vi "5492_TalonDriveTrainPID.vi"(0 "P Left":dbl, 1 "I Left":dbl, 2 "D Left":dbl, 3 "P Right":dbl, 4 "I Right":dbl, 5 "D Right":dbl) -> (14 "RobotDriveDevRef":T1={"DevStatus"={"status"=FALSE, "code"=0, "source"=""}, "Motors[]"=[], "Square Inputs"=FALSE, "Max Output"=1.0})   [LabVIEW 2017]
uses:
  <vilib>/Rock Robotics/WPI/RobotDrive/WPI_RobotDriveDevRef.ctl
  <vilib>/Rock Robotics/WPI/MotorControl/WPI_MotorControlDeviceRef.ctl
  <vilib>/Rock Robotics/WPI/MotorControl/WPI_MotorControlType.ctl
  <vilib>/Rock Robotics/SystemInterfaces/DIO/FPGA_DIOPWMChannel.ctl
  <vilib>/Rock Robotics/WPI/PWM/WPI_PWMDeadband.ctl
  <vilib>/Rock Robotics/SystemInterfaces/DIO/FPGA_DIOChannel.ctl
  5492_WPI_RobotDriveMotorSelectorEnum.ctl
  Public/Documents/Cross The Road Electronics/Phoenix-LabVIEW/Motor Controller/Controls/CTRE_Phoenix_MotorControl_FeedbackDevice.ctl
  <vilib>/Rock Robotics/WPI/Utilities/WPI_GetSetVariantRefNum.vi
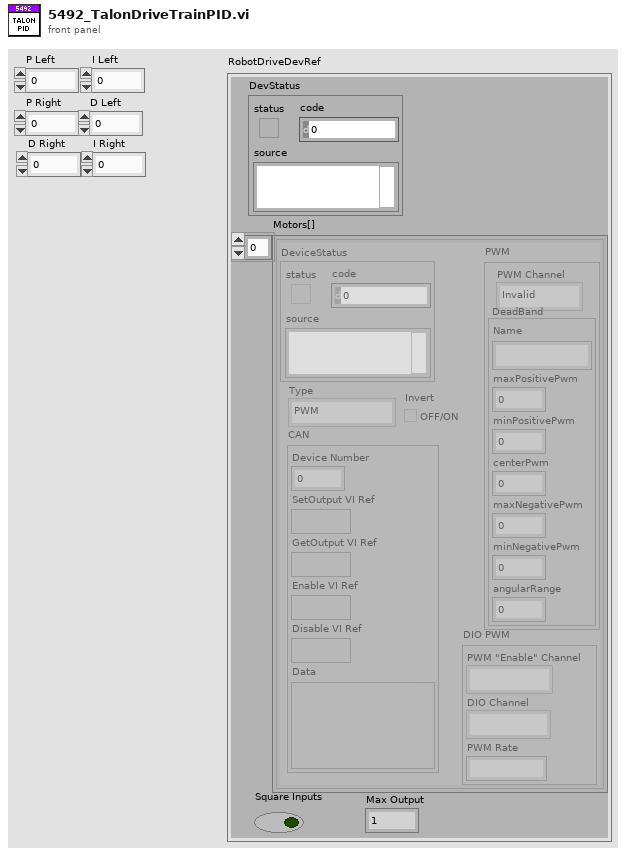
[diagram p1: front panel]
types:
  T1 = typedef "WPI_RobotDriveDevRef.ctl" = cluster{"DevStatus":errorcluster, "Motors[]":T2[], "Square Inputs":bool, "Max Output":dbl}
  T2 = typedef "WPI_MotorControlDeviceRef.ctl" = cluster{"DeviceStatus":errorcluster, "Type":T3, "PWM":cluster{"PWM Channel":T4, "DeadBand":T5}, "CAN":cluster{"Device Number":u8, "SetOutput VI Ref":variant, "GetOutput VI Ref":variant, "Enable VI Ref":variant, "Disable VI Ref":variant, "Data":variant}, "Invert":bool, "DIO PWM":cluster{"PWM \"Enable\" Channel":T4, "DIOChannel":T6, "PWM Rate":dbl}}
  T3 = typedef "WPI_MotorControlType.ctl" = enum16{"PWM", "CAN", "DIO PWM"}
  T4 = typedef "FPGA_DIOPWMChannel.ctl" = enum8{"PWM 0", "PWM 1", "PWM 2", "PWM 3", "PWM 4", "PWM 5", "PWM 6", "PWM 7", "PWM 8", "PWM 9", "PWM MXP 0", "PWM MXP 1", "PWM MXP 2", "PWM MXP 3", "PWM MXP 4", "PWM MXP 5", "PWM MXP 6", "PWM MXP 7", "PWM MXP 8", "PWM MXP 9", "Invalid"}
  T5 = typedef "WPI_PWMDeadband.ctl" = cluster{"Name":string, "maxPositivePwm":i32, "minPositivePwm":i32, "centerPwm":i32, "maxNegativePwm":i32, "minNegativePwm":i32, "angularRange":u16}
  T6 = typedef "FPGA_DIOChannel.ctl" = enum8{"DIO 0", "DIO 1", "DIO 2", "DIO 3", "DIO 4", "DIO 5", "DIO 6", "DIO 7", "DIO 8", "DIO 9", "DIO MXP 0", "DIO MXP 1", "DIO MXP 2", "DIO MXP 3", "DIO MXP 4", "DIO MXP 5", "DIO MXP 6", "DIO MXP 7", "DIO MXP 8", "DIO MXP 9", "DIO MXP 10", "DIO MXP 11", "DIO MXP 12", "DIO MXP 13", "DIO MXP 14", "DIO MXP 15", "SPI Port CS1", "SPI Port CS2", "SPI Port CS3", "SPI Port MISO", "SPI Port MOSI", "Invalid"}
  T7 = typedef "CTRE_Phoenix_MotorControl_FeedbackDevice.ctl" = i8
  T8 = typedef "5492_WPI_RobotDriveMotorSelectorEnum.ctl" = enum16{"Front left motor", "Front right motor"}
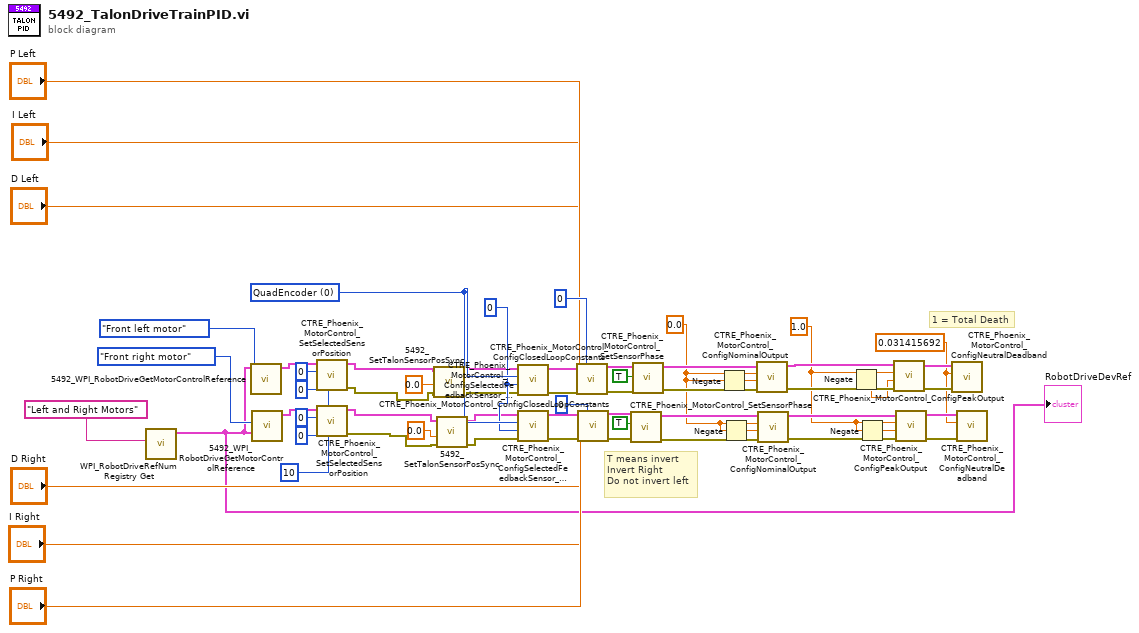
[diagram p0: block diagram]
diagram:
  w3 = 0.031415692 ("Percent Deadband")
  w11 = 0.0 ("Forward Nominal Percent Output")
  w12 = 1.0 ("Forward Peak Percent Output")
  w37 = u32 10 ("timeoutMs")
  w56 = 0 ("pidLoopIdx")
  w57 = T7 0 items=["None"=-1, "QuadEncoder"=0, "Analog"=2, "Tachometer"=4, "Pulse Width Encoded Position"=8, "Sensor Sum (S0 + S1)"=9, "Sensor Difference (D0 - D1)"=10, "Remote Source 0"=11, "Remote Source 1"=12, "Software Emulated"=15] ("Feedback Device")
  # "1 = Total Death"
  # "T means invert\nInvert Right\nDo not invert left"
  n1 = call <vilib>:"WPI_RobotDriveRefNum Registry Get.vi"("refnum name"="Left and Right Motors") -> ("RobotDriveDevRef"=w2:T1)  [unwired: 1 in, 9 out]
  "RobotDriveDevRef" <- w2
  n2 = call "5492_WPI_RobotDriveGetMotorControlReference.vi"("MotorIndex"=5492_WPI_RobotDriveMotorSelectorEnum."Front left motor", "RobotDriveDevRef"=w2) -> ("MotorControlDeviceRef"=w43:T2)  [unwired: 9 out]
  n3 = call "5492_WPI_RobotDriveGetMotorControlReference.vi"("MotorIndex"=5492_WPI_RobotDriveMotorSelectorEnum."Front right motor", "RobotDriveDevRef"=w2) -> ("MotorControlDeviceRef"=w40:T2)  [unwired: 9 out]
  n4 = call "CTRE_Phoenix_MotorControl_SetSelectedSensorPosition.vi"("timeoutMs"=w37, "pidLoopIdx"=u32 0, "New Sensor Position"=0, "PhoenixMotorControlDevRef"=w43) -> ("error out"=w30:errorcluster, "PhoenixMotorControlDevRef"=w35:T2)  [unwired: 6 in]
  n5 = call "CTRE_Phoenix_MotorControl_SetSelectedSensorPosition.vi"("timeoutMs"=w37, "pidLoopIdx"=u32 0, "New Sensor Position"=0, "PhoenixMotorControlDevRef"=w40) -> ("error out"=w29:errorcluster, "PhoenixMotorControlDevRef"=w33:T2)  [unwired: 6 in]
  n6 = call "5492_SetTalonSensorPosSync.vi"("error in (no error)"=w30, "Pos"=0.0 ("Output"), "CAN Talon SRX Ref In"=w35) -> ("error out"=w31:errorcluster, "CAN Talon SRX Ref Out"=w34:T2)  [unwired: 7 in]
  n7 = call "5492_SetTalonSensorPosSync.vi"("error in (no error)"=w29, "Pos"=0.0 ("Output"), "CAN Talon SRX Ref In"=w33) -> ("error out"=w28:errorcluster, "CAN Talon SRX Ref Out"=w32:T2)  [unwired: 7 in]
  n8 = call "CTRE_Phoenix_MotorControl_ConfigSelectedFeedbackSensor_Enhanced.vi"("error in (no error)"=w31, "pidLoopIdx"=w56, "Feedback Device"=w57, "PhoenixMotorControlDevRef"=w34) -> ("error out"=w54:errorcluster, "PhoenixMotorControlDevRef"=w55:T2)  [unwired: 6 in]
  n9 = call "CTRE_Phoenix_MotorControl_ConfigSelectedFeedbackSensor_Enhanced.vi"("error in (no error)"=w28, "pidLoopIdx"=w56, "Feedback Device"=w57, "PhoenixMotorControlDevRef"=w32) -> ("error out"=w52:errorcluster, "PhoenixMotorControlDevRef"=w53:T2)  [unwired: 6 in]
  n10 = call "CTRE_Phoenix_MotorControl_ConfigClosedLoopConstants.vi"("PhoenixMotorControlDevRef"=w55, "slotIdx"=0, "P"="P Left", "I"="I Left", "D"="D Left", "error in (no error)"=w54) -> ("PhoenixMotorControlDevRef"=w49:T2, "error out"=w48:errorcluster)  [unwired: 8 in]
  n11 = call "CTRE_Phoenix_MotorControl_ConfigClosedLoopConstants.vi"("PhoenixMotorControlDevRef"=w53, "slotIdx"=0, "P"="P Right", "I"="I Right", "D"="D Right", "error in (no error)"=w52) -> ("PhoenixMotorControlDevRef"=w50:T2, "error out"=w51:errorcluster)  [unwired: 8 in]
  n12 = call "CTRE_Phoenix_MotorControl_SetSensorPhase.vi"("error in (no error)"=w51, "PhaseSensor"=TRUE, "PhoenixMotorControlDevRef"=w50) -> ("error out"=w14:errorcluster, "PhoenixMotorControlDevRef"=w17:T2)  [unwired: 7 in]
  n13 = call "CTRE_Phoenix_MotorControl_SetSensorPhase.vi"("error in (no error)"=w48, "PhaseSensor"=TRUE, "PhoenixMotorControlDevRef"=w49) -> ("error out"=w18:errorcluster, "PhoenixMotorControlDevRef"=w21:T2)  [unwired: 7 in]
  n14 = Negate(x=w11) -> (-x=w13:dbl)
  n15 = Negate(x=w11) -> (-x=w10:dbl)
  n16 = call "CTRE_Phoenix_MotorControl_ConfigNominalOutput.vi"("error in (no error)"=w18, "Reverse Nominal Percent Output"=w13, "Forward Nominal Percent Output"=w11, "PhoenixMotorControlDevRef"=w21) -> ("error out"=w19:errorcluster, "PhoenixMotorControlDevRef"=w20:T2)  [unwired: 6 in]
  n17 = call "CTRE_Phoenix_MotorControl_ConfigNominalOutput.vi"("error in (no error)"=w14, "Reverse Nominal Percent Output"=w10, "Forward Nominal Percent Output"=w11, "PhoenixMotorControlDevRef"=w17) -> ("error out"=w15:errorcluster, "PhoenixMotorControlDevRef"=w16:T2)  [unwired: 6 in]
  n18 = Negate(x=w12) -> (-x=w8:dbl)
  n19 = Negate(x=w12) -> (-x=w9:dbl)
  n20 = call "CTRE_Phoenix_MotorControl_ConfigPeakOutput.vi"("error in (no error)"=w19, "Reverse Peak Percent Output"=w8, "Forward Peak Percent Output"=w12, "PhoenixMotorControlDevRef"=w20) -> ("error out"=w4:errorcluster, "PhoenixMotorControlDevRef"=w5:T2)  [unwired: 6 in]
  n21 = call "CTRE_Phoenix_MotorControl_ConfigPeakOutput.vi"("error in (no error)"=w15, "Reverse Peak Percent Output"=w9, "Forward Peak Percent Output"=w12, "PhoenixMotorControlDevRef"=w16) -> ("error out"=w6:errorcluster, "PhoenixMotorControlDevRef"=w7:T2)  [unwired: 6 in]
  n22 = call "CTRE_Phoenix_MotorControl_ConfigNeutralDeadband.vi"("error in (no error)"=w4, "Percent Deadband"=w3, "PhoenixMotorControlDevRef"=w5) -> ()  [unwired: 7 in, 2 out]
  n23 = call "CTRE_Phoenix_MotorControl_ConfigNeutralDeadband.vi"("error in (no error)"=w6, "Percent Deadband"=w3, "PhoenixMotorControlDevRef"=w7) -> ()  [unwired: 7 in, 2 out]
